vi "Get angle.vi"(10 "Circle details":T1, 11 "Edge location":cluster{"X":sgl, "Y":sgl}) -> (3 "Numeric":sgl)   [LabVIEW 2019]
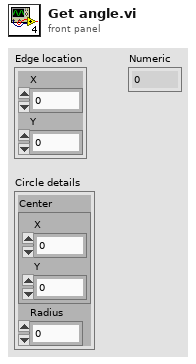
[diagram p1: front panel]
types:
  T1 = cluster{"Center":cluster{"X":sgl, "Y":sgl}, "Radius":dbl}
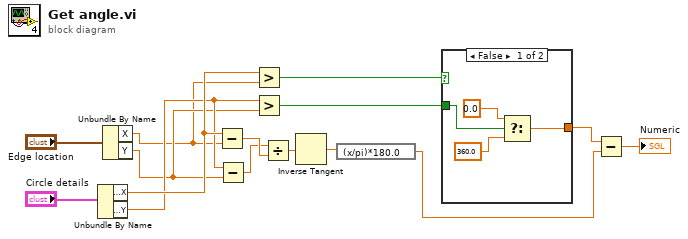
[diagram p0: block diagram]
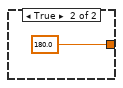
[diagram p2: hidden frame]
diagram:
  n1 = Unbundle By Name("Circle details") -> ("Center.X"=w6:sgl, "Center.Y"=w4:sgl)
  n2 = Unbundle By Name("Edge location") -> ("X"=w1:sgl, "Y"=w3:sgl)
  n3 = Subtract(x=w6, y=w1) -> (x-y=w10:sgl)
  n4 = Subtract(x=w4, y=w3) -> (x-y=w9:sgl)
  n5 = Greater?(x=w6, y=w1) -> (0:w5:bool)
  n6 = Greater?(x=w4, y=w3) -> (0:w2:bool)
  n7 = Divide(x=w9, y=w10) -> (x/y=w11:sgl)
  n8 = Inverse Tangent(1:w11) -> (0:w12:sgl)
  n9 = expression code="(x/pi)*180.0" ("radians to degrees")(w12) -> (w13:sgl)
  n10 = case shown="False" w5 {
    tunnel: [w19 sgl 180.0 ("x")] -> w14
    tunnel: w2 -> [w18 _]
    frame False {
      n11 = Select(t=0.0, s=w18, f=360.0) -> (s? t:f=w19:dbl)
    }
    frame True {
    }
  }
  n12 = Subtract(x=w14, y=w13) -> (x-y=→"Numeric":dbl)
